vi "BeamFeedForward.vi"(7 "Reset":bool=TRUE, 8 "input valid":bool=TRUE, 9 "beam enabled":bool=TRUE, 11 "Data in":fxp<+/-,16,14>[](array[numeric])=[0.0, 0.0]) -> (0 "output valid":bool, 3 "Data out":fxp<+/-,16,14>[](array[numeric]))   [LabVIEW 2013]
doc: "Calculates various combinations on I_in, Q_in and cos(fi) and sin(fi) to be used later to delay the output signal"
uses:
  <vilib>/rvi/Memory/Memory_Emulation/nirvimemoryFastEmulationFpgaImpl.vi
  <instcachedir>/0/nirvimemoryFastEmulationFpgaImpl_5FBAB50466BC4C939F684F8805638BFC.lvgen/nirvimemoryFastEmulationFpgaImpl_5FBAB50466BC4C939F684F8805638BFC_001.vi
  <vilib>/rvi/DataTransferAndStorage/Container/Common/niFpgaContainerGetUniqueNameForEmu.vi
  <vilib>/rvi/Memory/Memory_Emulation/nirvimemoryFastEmulation.vi
  <vilib>/rvi/Memory/Memory_Emulation/nirvimemoryEmulation.vi
  <vilib>/rvi/DataTransferAndStorage/Container/XNode/niFpgaContainer.xnode
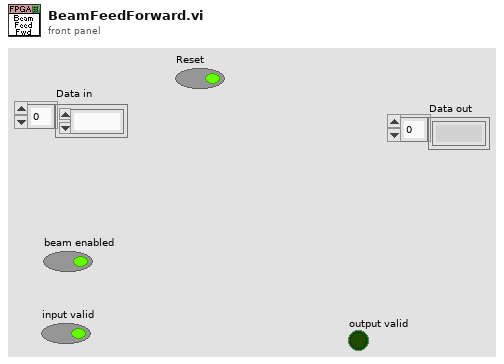
[diagram p1: front panel]
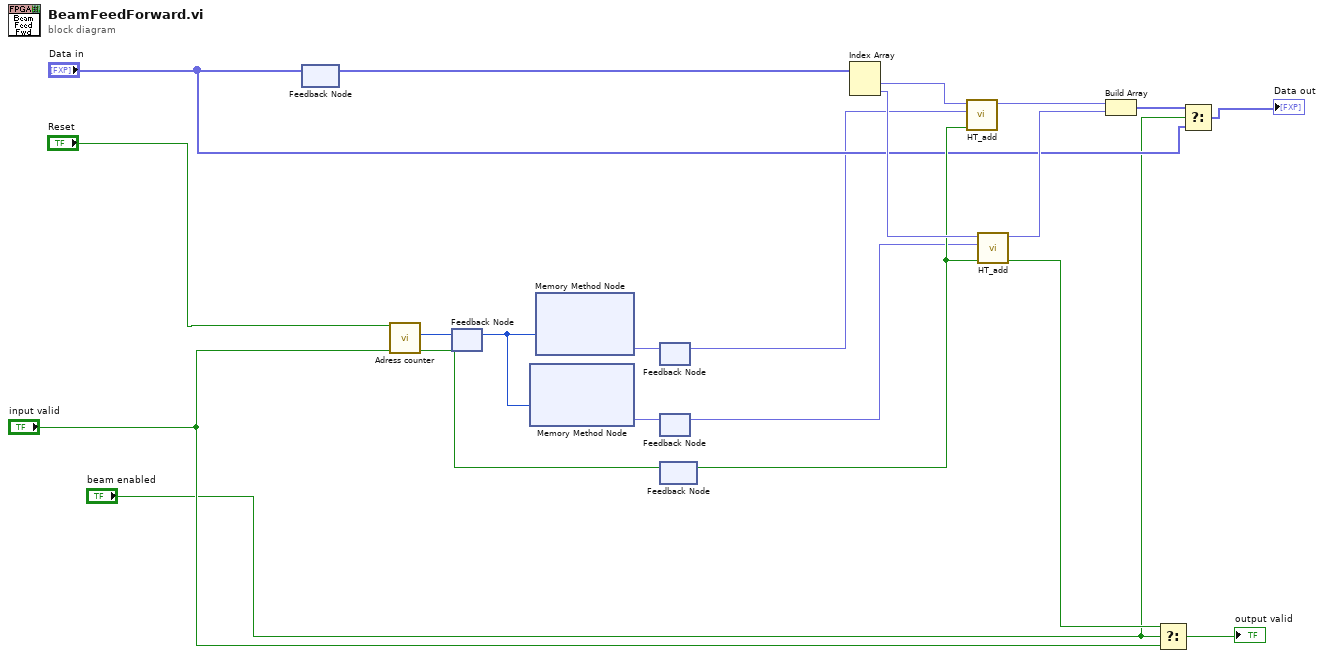
[diagram p0: block diagram]
diagram:
  n1 = feedback #1() -> (w20:fxp<+/-,16,14>[])  [unwired: 1 in]
  n2 = feedback-in #1("Data in") -> ()
  n3 = call "Adress counter.vi"("input valid"="input valid", "Reset"="Reset") -> ("output valid"=w21:bool, "Address"=w2:u32)  [unwired: 8 in]
  n4 = feedback #2() -> (w1:u32)  [unwired: 1 in]
  n5 = feedback-in #2(w2) -> ()
  n6 = xnode ("Memory Method Node")("Address"=w1) -> ("Data"=w3:fxp<+/-,16,14>)  [unwired: 1 in, 1 out]
  n7 = xnode ("Memory Method Node")("Address"=w1) -> ("Data"=w4:fxp<+/-,16,14>)  [unwired: 1 in, 1 out]
  n8 = feedback #3() -> (w6:fxp<+/-,16,14>)  [unwired: 1 in]
  n9 = feedback-in #3(w4) -> ()
  n10 = feedback #4() -> (w5:fxp<+/-,16,14>)  [unwired: 1 in]
  n11 = feedback-in #4(w3) -> ()
  n12 = feedback #5() -> (w17:bool)  [unwired: 1 in]
  n13 = feedback-in #5(w21) -> ()
  n14 = Index Array(array=w20) -> (element #1=w7:fxp<+/-,16,14>, element #2=w18:fxp<+/-,16,14>)  [unwired: 2 in]
  n15 = call "HT_add.vi"("input valid"=w17, "y"=w6, "x"=w7) -> ("x+y"=w16:fxp<+/-,16,14>)  [unwired: 7 in, 1 out]
  n16 = call "HT_add.vi"("input valid"=w17, "y"=w5, "x"=w18) -> ("output valid"=w14:bool, "x+y"=w15:fxp<+/-,16,14>)  [unwired: 7 in]
  n17 = Build Array(w16, w15) -> (w11:fxp<+/-,16,14>[])
  n18 = Select(t=w14, s="beam enabled", f="input valid") -> (s? t:f=→"output valid":bool)
  n19 = Select(t=w11, s="beam enabled", f="Data in") -> (s? t:f=→"Data out":fxp<+/-,16,14>[])
